vi "AlliGator Select Phasor Calibration v3.vi"(4 "Calibration Map MD5 Digest":string, 6 "Current Data Set (-1: single)":i32=-1, 7 "ROI Center (Default: undefined)":cluster{"X":i32, "Y":i32}={"X"=2147483647, "Y"=2147483647}, 8 "Error In":errorcluster, 9 "Phasor Calibration Map":T3={"Phasor Frequency"=80000000.0, "Calibration Lifetime"=1e-09, "ROI Centers"=[], "ROI Descriptors"=[], "Map Resolution X"=0, "Map Resolution Y"=0, "z Array"=[]} {"ROI Descriptors"."Contours"."Type" items=["No Selection", "Point", "Line", "Rectangle", "Oval", "Polygon", "Freehand Region", "Annulus", "Unused2", "Unused3", "Broken Line", "Freehand Line", "Rotated Rectangle"]}, 10 "Calibration Phasor Series":T6, 11 "Calibration Phasor":T5={"m"=1.0, "phi"=0.0, "Phasor Frequency"=0.0, "Reference Lifetime"=0.0}) -> (0 "Error Out":errorcluster, 1 "Phasor Calibration Map Characteristics":T1={"Phasor Frequency"=80000000.0, "Calibration Lifetime"=1e-09, "Map Resolution X"=0, "Map Resolution Y"=0, "Empty Map"=FALSE}, 2 "Calibration Type Used":T2, 3 "Calibration Phasor":T5)   [LabVIEW 2021, in "AlliGator Phasor Calibration.lvlib"]
doc: "Picks the appropriate Phasor Calibration, depending on the <B>ROI Center</B> and <B>Current Data Set</B> and phasor calibration options (single calibration, series or map)."
uses:
  AlliGator Phasor Calibration.lvlib
  Phasor/Phasor Reference Series.ctl
  Phasor/Calibration Phasor (m, phi).ctl
  Phasor/Phasor Calibration Map v2.ctl
  Phasor/Phasor Calibration Type.ctl
  Phasor/Phasor Calibration Map Characteristics.ctl
  AlliGator Settings List.ctl
  Phasor/Phasor.lvlib
  AlliGator Settings.lvlib
panel:
  # "see the AlliGator License on the block diagram (Ctrl+E or Window:Show Block Diagram)"
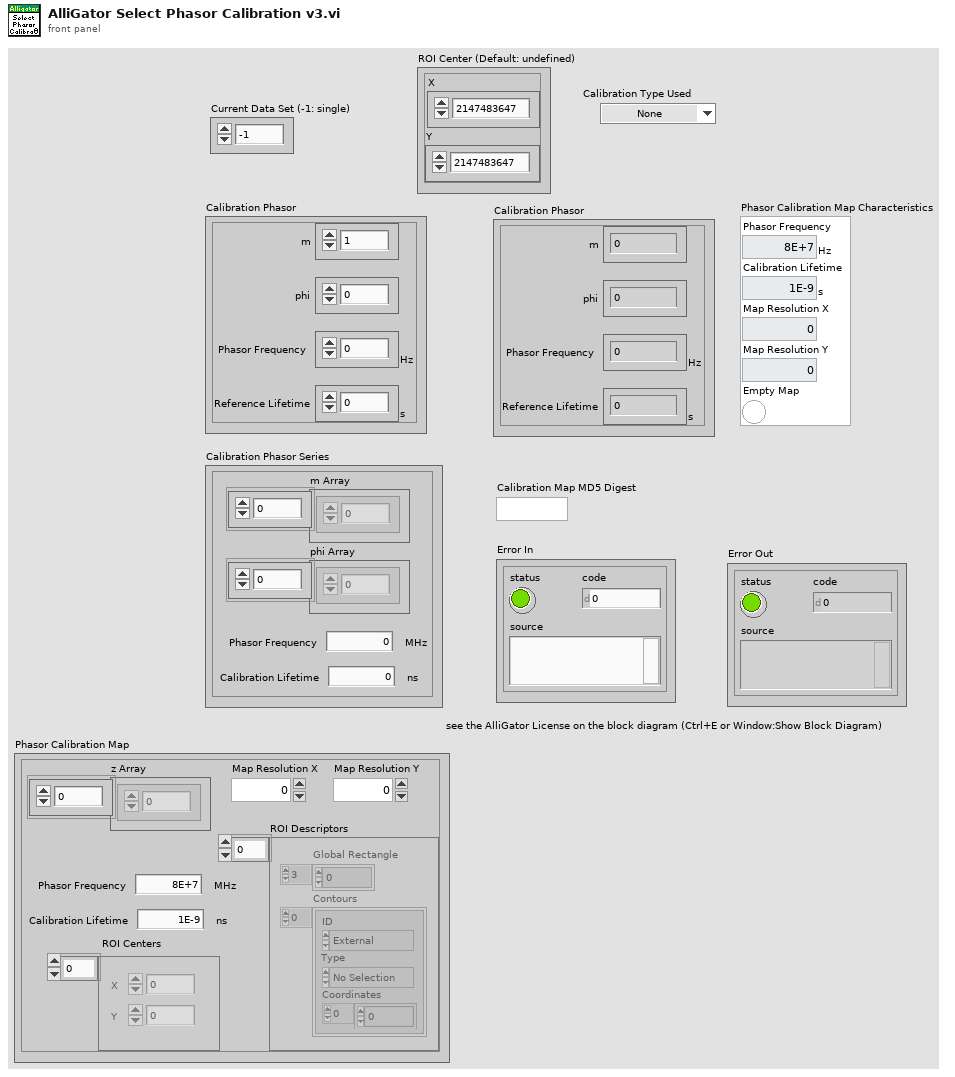
[diagram p1: front panel]
types:
  T1 = typedef "Phasor.lvlib/Phasor Calibration Map Characteristics.ctl" = cluster{"Phasor Frequency":dbl[unit], "Calibration Lifetime":dbl[unit], "Map Resolution X":i32, "Map Resolution Y":i32, "Empty Map":bool}
  T2 = typedef "Phasor.lvlib/Phasor Calibration Type.ctl" = enum16{"None", "Single Phasor", "Phasor Series", "Phasor Map"}
  T3 = typedef "Phasor.lvlib/Phasor Calibration Map v2.ctl" = cluster{"Phasor Frequency":dbl[unit], "Calibration Lifetime":dbl[unit], "ROI Centers":cluster{"X":i32, "Y":i32}[], "ROI Descriptors":T4[], "Map Resolution X":i32, "Map Resolution Y":i32, "z Array":cdb[]}
  T4 = typedef "ROI Descriptor" = cluster{"Global Rectangle":i32[], "Contours":cluster{"ID":enum32{"External", "Internal"}, "Type":u32, "Coordinates":i32[]}[]}
  T5 = typedef "Phasor.lvlib/Calibration Phasor (m, phi).ctl" = cluster{"m":dbl, "phi":dbl, "Phasor Frequency":dbl[unit], "Reference Lifetime":dbl[unit]}
  T6 = typedef "Phasor.lvlib/Phasor Reference Series.ctl" = cluster{"m Array":dbl[], "phi Array":dbl[], "Phasor Frequency":dbl[unit], "Calibration Lifetime":dbl[unit]}
  T7 = typedef "AlliGator Settings.lvlib/AlliGator Settings List.ctl" = enum16{"GUI:Visible Settings Tab", "GUI:Last Run Version", "Source Image:Use Image Histogram for Contrast", "Source Image:Low Count Pixels Rejection Options", "Source Image:High Count Pixels Rejection Options", "Source Image:Use Image Brightness", "Source Image:Blend Overlay with Image Background", "Source Image:Use Fixed ROI Diameter", "Source Image:ROI Diameter", "Source Image:ROI Center Color", "Source Image:Peak Threshold", "Source Image:Intensity Threshold", "Source Image:Image Binning Options", "Source Image:Image Smoothing Options", "Source Image:Image Histogram Active", "Source Image:Invert Binary Mask", "Source Image:Hot Pixel Removal", "Source Image:Overlay Analyzed ROI Center", "Source Image:Auto-Adjust Contrast", "Source Image:Histogram Lower Percentile", "Source Image:Histogram Upper Percentile", "Source Image:Save Source Image", "Source Image:Scale Bar Options", "Source Image:Image Resolution (Pixel Size)", "Source Image:Flatfield Correction", "Data Information:Gate Width", "Data Information:Nanotime Gate Separation", "Data Information:Macrotime Gate Separation", "Data Information:Gate Step", "Data Information:# Gates", "Data Information:Gate Image Exposure", "Data Information:Gate Image Integration", "Data Information:Gates to Skip", "Data Information:Gates to Keep", "Data Information:Define Gates to", "Data Information:Channel Name", "Data Information:Available Channel Names", "Data Information:Channel Arithmetic", "Data Information:Background File Subtraction", "Data Information:Background File", "Data Information:Background Scaling Factor", "Data Information:Background Pile-up Correction", "Data Information:Background Pixel Well Capacity", "Data Information:Laser Period", "Data Information:SYNC Period", "Data Information:Pile-up Correction", "Data Information:Pixel Well Capacity", "Data Information:Dataset Scaling Factor", "Fluorescence Decay_Decay Pre-Processing:Reverse Gates", "Fluorescence Decay_Decay Pre-Processing:Verbose Decay Pre-Processing", "Fluorescence Decay_Decay Pre-Processing:Use Decay Pre-Processing", "Fluorescence Decay_Decay Pre-Processing:Background Subtraction", "Fluorescence Decay_Decay Pre-Processing:Background Definition Range", "Fluorescence Decay_Decay Pre-Processing:Baseline Subtraction Method", "Fluorescence Decay_Decay Pre-Processing:Operations Order", "Fluorescence Decay_Decay Pre-Processing:Smoothing Parameter", "Fluorescence Decay_Decay Pre-Processing:Shift Decay", "Fluorescence Decay_Decay Pre-Processing:Decay Shift Parameters", "Fluorescence Decay_Decay Pre-Processing:Fold Decay", "Fluorescence Decay_Decay Pre-Processing:# Folds", "Fluorescence Decay_Decay Pre-Processing:1-Normalize Decay", "Fluorescence Decay_Decay Pre-Processing:[0-1]-Normalize Decay", "Fluorescence Decay_Decay Pre-Processing:Smoothen Decay", "Fluorescence Decay_Decay Pre-Processing:Extrapolate Decay", "Fluorescence Decay_Decay Pre-Processing:Use Periodicity", "Fluorescence Decay_Decay Pre-Processing:Use Cursors", "Fluorescence Decay_Decay Pre-Processing:Tail Fraction", "Fluorescence Decay_Decay Pre-Processing:Head Fraction", "Fluorescence Decay_Decay Pre-Processing:Additional Points", "Fluorescence Decay_Decay Pre-Processing:Straighten Decay", "Fluorescence Decay_Decay Pre-Processing:Constant Background", "Fluorescence Decay_Decay Pre-Processing:Pixel-Normalize Decay", "Fluorescence Decay_Advanced Analysis:Extract IRF instead of Decay", "Fluorescence Decay_Advanced Analysis:IRF Extraction Options", "Fluorescence Decay_Advanced Analysis:IRF Optimization Options", "Fluorescence Decay_Advanced Analysis:Square Pulse Options", "Fluorescence Decay_Advanced Analysis:IRF Order", "Fluorescence Decay_Advanced Analysis:IRF Time Constants", "Fluorescence Decay_Advanced Analysis:Wavelet Analysis Options", "Fluorescence Decay_Advanced Analysis:Average Lifetime Options", "Fluorescence Decay_Fit Options:Fit Options", "Fluorescence Decay_Fit Options:Use Legacy Fitting Approach", "Fluorescence Decay_Fit Options:Use Data Information Laser Period", "Fluorescence Decay_Fit Parameters:Displayed Fit Parameters", "Fluorescence Decay_Fit Parameters:Fit Parameter Constraints", "Fluorescence Decay_Fit Parameters:Export Tabulated Results", "Fluorescence Decay_Fit Parameters:MLE Baseline Offset Type", "Fluorescence Decay_Fit Parameters:MLE Baseline Offset", "Fluorescence Decay_Fit Parameters:Guess Parameter Names", "Fluorescence Decay_Fit Parameters:Guess Parameter Values", "Fluorescence Decay_Fit Parameters:Guess Parameters Options", "Fluorescence Decay_Styles:Show Last Decay Only", "Fluorescence Decay_Styles:Decay Graph Color Array", "Fluorescence Decay:Decay Graph Active", "Fluorescence Decay Statistics:Min Peak Value", "Fluorescence Decay Statistics:Reject Low Decay Peak Pixels", "Fluorescence Decay Statistics:Reject High Decay Peak Pixels", "Fluorescence Decay Statistics:Max Peak Value", "Time Traces:Use File Timestamp", "Time Traces:Time Step", "Time Traces:Use Intensity Correction File", "Time Traces:Intensity Correction File", "Phasor Plot:Phasor Plot Smoothing Options", "Phasor Plot:Phasor Plot Size", "Phasor Plot:Phasor Plot Graphics Options", "Phasor Plot:Cumulative Phasor Plot", "Phasor Plot:Use Phasor Brightness", "Phasor Plot:Blend Overlay with Phasor Background", "Phasor Plot:Save Phasor Plot", "Phasor Plot:Show References", "Phasor Plot:Phasor Ratio Decay Range", "Phasor Plot:Exponential Fading", "Phasor Plot:Phasor Ratio Reference Colors", "Phasor Plot:Reference Radius", "Phasor Plot:Show Color Map Vertices", "Phasor Plot:Phasor Plot Active", "Phasor Plot:Phasor Ratio Color Map Type", "Phasor Plot:Phasor Ratio Color Map", "Phasor Plot:Phasor Ratio Display Range", "Phasor Plot:Selected Image ROI(s)", "Phasor Plot:All Image ROIs", "Phasor Plot:Selected Phasor Plot ROI(s)", "Phasor Plot:All Phasor Plot ROIs", "Phasor Plot:Phasor Ratio Color-Coded Quantity", "Phasor Plot:Store Phasor Harmonics", "Phasor Plot:Draw Reference Segment", "Phasor Plot:User-Defined Quantity", "Phasor Graph:Phasor Frequency", "Phasor Graph:Phasor Ratio Type", "Phasor Graph:Pixel-level Phasor Computation", "Phasor Graph:Save Phasor Graph", "Phasor Graph:Phasor Graph Active", "Phasor Graph:Phasor SDV Options", "Phasor Calibration:Use Backup Calibration if needed", "Phasor Graph:Define Shortest Lifetime as", "Phasor Calibration:Backup Calibration Type", "Phasor Calibration:Calibration Type", "Phasor Calibration:Calibration Lifetime", "Phasor Calibration:Calibration Map Algorithm", "Single-Exponential Phasor Locus (SEPL):Gate Parameters", "Single-Exponential Phasor Locus (SEPL):User-defined Gate", "Single-Exponential Phasor Locus (SEPL):User-defined IRF", "Single-Exponential Phasor Locus (SEPL):Phasor Parameters", "Single-Exponential Phasor Locus (SEPL):Decay & IRF Parameters", "Single-Exponential Phasor Locus (SEPL):Display Parameters", "Lifetime Analysis:Decay Analysis Parameters", "Lifetime Analysis:Lifetime Map Active", "Plugins:Python Settings", "Miscellaneous:Verbose Mode", "Miscellaneous:Beep after Script", "Miscellaneous:Saved Image File Format", "Miscellaneous:Exported Gate Image Settings", "Miscellaneous:Include Loading in Timing", "Miscellaneous:Verbose Settings Mode", "Miscellaneous:Histogram Options", "Miscellaneous:Beep on Error", "Miscellaneous:# Logical Processors Used", "Miscellaneous:ROI Description Max Characters", "Miscellaneous:Verbose Error Mode", "Miscellaneous:Transparent Mask Color"}
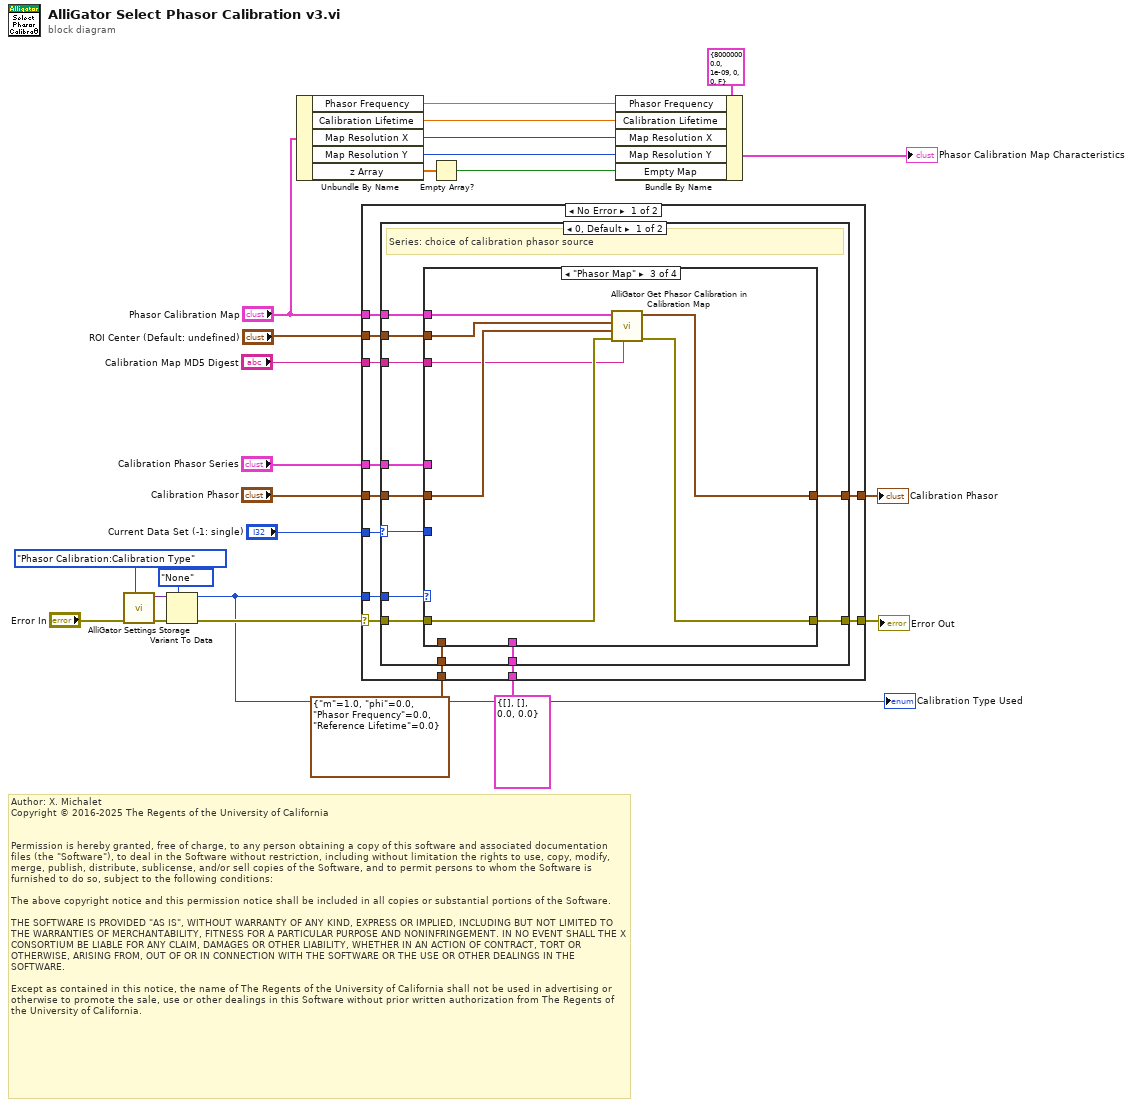
[diagram p0: block diagram]
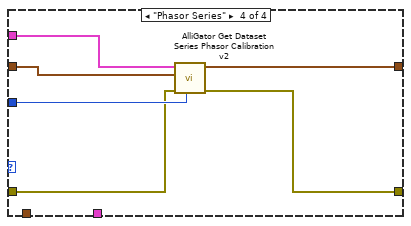
[diagram p4: hidden frame]
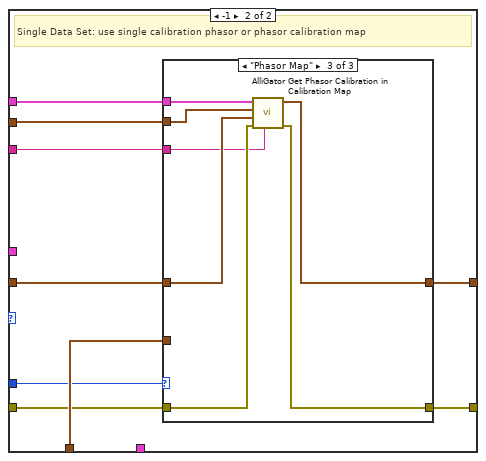
[diagram p5: hidden frame]
diagram:
  # "Author: X. Michalet\nCopyright © 2016-2025 The Regents of the University of California\n \n\nPermission is hereby granted, free of charge, to any person obtaining a copy of this software and associated documentation files (the \"Software\"), to deal in the Software without restriction, including without limitation the rights to use, copy, modify, merge, publish, distribute, sublicense, and/or sell copies of the Software, and to permit persons to whom the Software is furnished to do so, subject to the following conditions:\n\nThe above copyright notice and this permission notice shall be included in all copies or substantial portions of the Software.\n\nTHE SOFTWARE IS PROVIDED \"AS IS\", WITHOUT WARRANTY OF ANY KIND, EXPRESS OR IMPLIED, INCLUDING BUT NOT LIMITED TO THE WARRANTIES OF MERCHANTABILITY, FITNESS FOR A PARTICULAR PURPOSE AND NONINFRINGEMENT. IN NO EVENT SHALL THE X CONSORTIUM BE LIABLE FOR ANY CLAIM, DAMAGES OR OTHER LIABILITY, WHETHER IN AN ACTION OF CONTRACT, TORT OR OTHERWISE, ARISING FROM, OUT OF OR IN CONNECTION WITH THE SOFTWARE OR THE USE OR OTHER DEALINGS IN THE SOFTWARE.\n\nExcept as contained in this notice, the name of The Regents of the University of California shall not be used in advertising or otherwise to promote the sale, use or other dealings in this Software without prior written authorization from The Regents of the University of California."
  n1 = call "AlliGator Settings Storage.vi"("AlliGator Settings List"=AlliGator_Settings_List."Phasor Calibration:Calibration Type", "Error In"="Error In") -> ("Error Out"=w13:errorcluster, "Variant Data out"=w14:variant)  [unwired: 8 in]
  n2 = Variant To Data(error in=w13, type=Phasor_Calibration_Type."None" ("Calibration Type"), Variant=w14) -> (data=w16:T2, error out=w18:errorcluster)
  "Calibration Type Used" <- w16
  n3 = Unbundle By Name("Phasor Calibration Map") -> ("Phasor Frequency"=w6:dbl[unit], "Calibration Lifetime"=w1:dbl[unit], "Map Resolution X"=w2:i32, "Map Resolution Y"=w3:i32, "z Array"=w5:cdb[])
  n4 = case shown="No Error" w18 {
    selector: w18 -> [w29 w87]
    tunnel: "Calibration Phasor Series" -> [w37 _]
    tunnel: "Calibration Phasor" -> [w36 _]
    tunnel: "Current Data Set (-1: single)" -> [w35 _]
    tunnel: [w34 w88] -> w22
    tunnel: T5 {"m"=1.0, "phi"=0.0, "Phasor Frequency"=0.0, "Reference Lifetime"=0.0} ("f") -> [w33 w88]
    tunnel: T6 {"m Array"=[], "phi Array"=[], "Phasor Frequency"=0.0, "Calibration Lifetime"=0.0} ("f") -> [w32 _]
    tunnel: "Phasor Calibration Map" -> [w31 _]
    tunnel: "ROI Center (Default: undefined)" -> [w30 _]
    tunnel: [w28 w87] -> w17
    tunnel: w16 -> [w27 _]
    tunnel: "Calibration Map MD5 Digest" -> [w26 _]
    frame No Error {
      n5 = case shown="0, Default" w35 {
        selector: w35 -> [w49 _]
        tunnel: w36 -> [w48 w75]
        tunnel: [w44 w73] -> w34
        tunnel: w37 -> [w46 _]
        tunnel: w33 -> [w47 w74]
        tunnel: w32 -> [w45 _]
        tunnel: w31 -> [w43 w72]
        tunnel: w30 -> [w42 w71]
        tunnel: w29 -> [w41 w70]
        tunnel: [w40 w69] -> w28
        tunnel: w27 -> [w39 w68]
        tunnel: w26 -> [w38 w67]
        frame 0, Default {
          # "Series: choice of calibration phasor source"
          n6 = case shown="\"Phasor Map\"" w39 {
            tunnel: w49 -> [_ _ _ w66]
            tunnel: w48 -> [_ w52 w55 w61]
            tunnel: w47 -> [w51 _ _ _]
            tunnel: w46 -> [_ _ _ w65]
            tunnel: w45 -> [_ _ _ _]
            tunnel: [w51 w52 w60 w64] -> w44
            tunnel: w43 -> [_ _ w59 _]
            tunnel: w42 -> [_ _ w58 _]
            tunnel: w41 -> [w50 w53 w57 w63]
            tunnel: [w50 w53 w56 w62] -> w40
            tunnel: w38 -> [_ _ w54 _]
            frame "None", Default {
            }
            frame "Single Phasor" {
            }
            frame "Phasor Map" {
              n7 = call "AlliGator Get Phasor Calibration in Calibration Map.vi"("Calibration Map MD5 Digest"=w54, "Error In"=w57, "Phasor Calibration in"=w55, "ROI Center"=w58, "Phasor Calibration Map"=w59) -> ("Error Out"=w56:errorcluster, "Phasor Calibration out"=w60:T5)  [unwired: 5 in]
            }
            frame "Phasor Series" {
              n8 = call "AlliGator Get Dataset Series Phasor Calibration v2.vi"("Dataset Series Index"=w66, "Error In"=w63, "Default Phasor Calibration"=w61, "Phasor Calibration Series"=w65) -> ("Error Out"=w62:errorcluster, "Phasor Calibration"=w64:T5)  [unwired: 6 in]
            }
          }
        }
        frame -1 {
          # "Single Data Set: use single calibration phasor or phasor calibration map"
          n9 = case shown="\"Phasor Map\"" w68 {
            tunnel: [w76 w79 w84] -> w73
            tunnel: w72 -> [_ _ w86]
            tunnel: w71 -> [_ _ w85]
            tunnel: w70 -> [w77 w78 w83]
            tunnel: [w77 w78 w82] -> w69
            tunnel: w75 -> [_ w79 w81]
            tunnel: w74 -> [w76 _ _]
            tunnel: w67 -> [_ _ w80]
            frame "None", Default {
            }
            frame "Single Phasor" {
            }
            frame "Phasor Map" {
              n10 = call "AlliGator Get Phasor Calibration in Calibration Map.vi"("Calibration Map MD5 Digest"=w80, "Error In"=w83, "Phasor Calibration in"=w81, "ROI Center"=w85, "Phasor Calibration Map"=w86) -> ("Error Out"=w82:errorcluster, "Phasor Calibration out"=w84:T5)  [unwired: 5 in]
            }
          }
        }
      }
    }
    frame Error {
    }
  }
  "Calibration Phasor" <- w22
  "Error Out" <- w17
  n11 = Empty Array?(array=w5) -> (empty?=w4:bool)
  n12 = Bundle By Name(cluster=T1 {"Phasor Frequency"=80000000.0, "Calibration Lifetime"=1e-09, "Map Resolution X"=0, "Map Resolution Y"=0, "Empty Map"=FALSE} ("Phasor Calibration Map Characteristics"), "Phasor Frequency"=w6, "Calibration Lifetime"=w1, "Map Resolution X"=w2, "Map Resolution Y"=w3, "Empty Map"=w4) -> (→"Phasor Calibration Map Characteristics":T1)
